vi "PH_Cont-601k_PSU.evt Call Set Mode.vi"(0 "i ref in":refnum<vi>, 1 "Instance name":string="N/A", 4 "Mode to set":T1, 5 "error in":errorcluster) -> (14 "i ref out":refnum<vi>, 19 "error out":errorcluster)   [LabVIEW 2014, in "PH_Cont-601k_PSU.lvlib"]
doc: "This VI calls an event by a simple call."
uses:
  PH_Cont-601k_PSU.lvlib
  PH_Cont-601k_PSU.Mode.ctl
  CSCore/CSSystem/CoreLib/CoreLib.int 2 byte array.vi
  CSCore/BaseProcess/BaseProcess.lvlib
  CSCore/CSSystem/CoreLib/CoreLib.lvlib
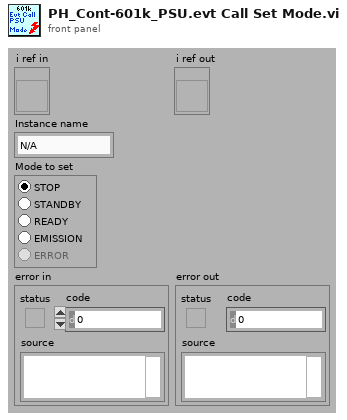
[diagram p1: front panel]
types:
  T1 = typedef "PH_Cont-601k_PSU.lvlib/PH_Cont-601k_PSU.Mode.ctl" = enum32{"STOP", "STANDBY", "READY", "EMISSION", "ERROR"}
  T2 = typedef "CoreDefs.rawDataType.ctl" = i8[]
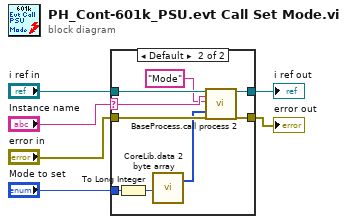
[diagram p0: block diagram]
diagram:
  n1 = case shown="Default" "Instance name" {
    selector: "Instance name" -> [_ w13]
    tunnel: [w7 w17] -> w6
    tunnel: "error in" -> [w7 w16]
    tunnel: [w8 w15] -> w3
    tunnel: "i ref in" -> [w8 w14]
    tunnel: "Mode to set" -> [_ w10]
    frame "", "N/A" {
    }
    frame Default {
      n2 = To Long Integer(number=w10) -> (32bit integer=w9:i32)
      n3 = call-poly "CoreLib.data 2 byte array.vi"("i32"=w9) -> ("byteArray out"=w11:T2)  [unwired: 18 in]
      n4 = call "BaseProcess.call process 2.vi"("i ref in"=w14, "Object"=w13, "Selector"="Mode", "Data"=w11, "error in (no error)"=w16) -> ("i ref out"=w15:refnum<vi>, "error out"=w17:errorcluster)  [unwired: 13 in]
    }
  }
  "error out" <- w6
  "i ref out" <- w3
